vi "Get Controler Scheme.vi"(8 "error in (no error)":errorcluster, 11 "JoystickDevRef":T2) -> (0 "error out":errorcluster, 2 "Control Values":T1, 3 "JoystickDevRef":T2)   [LabVIEW 2016]
doc: "This VI takes a controller's refnum and arranges it's input in a cluster based on it's control scheme.\n\nCreated by Team 4130 for use in the 2016-2017 FRC season"
uses:
  <vilib>/Rock Robotics/WPI/Joystick/WPI_JoystickDevRef.ctl
  <vilib>/Rock Robotics/WPI/Joystick/WPI_JoystickDeviceEnum.ctl
  <vilib>/Rock Robotics/Network Tables/NT Read Numeric Array.vi
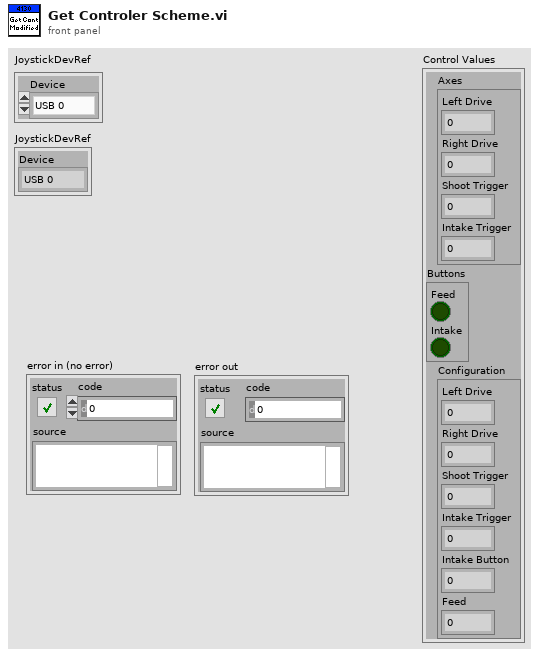
[diagram p1: front panel]
types:
  T1 = cluster{"Axes":cluster{"Left Drive":dbl, "Right Drive":dbl, "Shoot Trigger":dbl, "Intake Trigger":dbl}, "Buttons":cluster{"Feed":bool, "Intake":bool}, "Configuration":cluster{"Left Drive":i32, "Right Drive":i32, "Shoot Trigger":i32, "Intake Trigger":i32, "Intake Button":i32, "Feed":i32}}
  T2 = typedef "WPI_JoystickDevRef.ctl" = cluster{"Device":T3}
  T3 = typedef "WPI_JoystickDeviceEnum.ctl" = enum16{"USB 0", "USB 1", "USB 2", "USB 3", "USB 4", "USB 5"}
  T4 = cluster{"Left Drive":i32, "Right Drive":i32, "Shoot Trigger":i32, "Intake Trigger":i32, "Intake Button":i32, "Feed":i32}
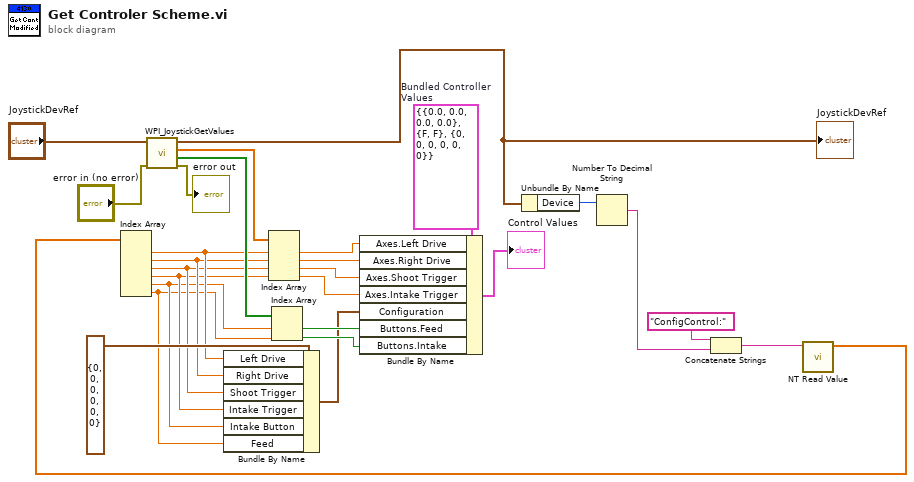
[diagram p0: block diagram]
diagram:
  w10 = T1 {"Axes"={"Left Drive"=0.0, "Right Drive"=0.0, "Shoot Trigger"=0.0, "Intake Trigger"=0.0}, "Buttons"={"Feed"=FALSE, "Intake"=FALSE}, "Configuration"={"Left Drive"=0, "Right Drive"=0, "Shoot Trigger"=0, "Intake Trigger"=0, "Intake Button"=0, "Feed"=0}}  # Bundled Controller Values
  n1 = call <vilib>:"WPI_JoystickGetValues.vi"("error in (no error)"="error in (no error)", "JoystickDevRef"="JoystickDevRef") -> ("error out"=→"error out":errorcluster, "Buttons"=w18:bool[], "Axes"=w17:dbl[], "JoystickDevRef"=w26:T2)  [unwired: 5 in, 1 out]
  "JoystickDevRef" <- w26
  n2 = Unbundle By Name(w26) -> ("Device"=w23:T3)
  n3 = Number To Decimal String(number=w23) -> (decimal integer string=w25:string)  [unwired: 1 in]
  n4 = Concatenate Strings("ConfigControl:", w25) -> (w27:string)
  n5 = call-poly <vilib>:"NT Read Value.vi"("Name"=w27) -> ("Numeric Array"=w9:dbl[])  [unwired: 9 in, 1 out]
  n6 = Index Array(array=w9) -> (element #1=w6:dbl, element #2=w5:dbl, element #3=w4:dbl, element #4=w3:dbl, element #5=w2:dbl, element #6=w1:dbl)  [unwired: 6 in]
  n7 = Bundle By Name(cluster=T4 {"Left Drive"=0, "Right Drive"=0, "Shoot Trigger"=0, "Intake Trigger"=0, "Intake Button"=0, "Feed"=0} ("Configuration"), "Left Drive"=w6, "Right Drive"=w5, "Shoot Trigger"=w4, "Intake Trigger"=w3, "Intake Button"=w2, "Feed"=w1) -> (w7:T4)
  n8 = Index Array(array=w17, index #1=w6, index #2=w5, index #3=w4, index #4=w3) -> (element #1=w11:dbl, element #2=w12:dbl, element #3=w13:dbl, element #4=w14:dbl)
  n9 = Index Array(array=w18, index #1=w2, index #2=w1) -> (element #1=w15:bool, element #2=w16:bool)
  n10 = Bundle By Name(cluster=w10, "Axes.Left Drive"=w11, "Axes.Right Drive"=w12, "Axes.Shoot Trigger"=w13, "Axes.Intake Trigger"=w14, "Configuration"=w7, "Buttons.Feed"=w15, "Buttons.Intake"=w16) -> (→"Control Values":T1)
